vi "Save As DataTable.vi"(6 "overwrite file if exist (true)?":bool=TRUE, 8 "error in (no error)":errorcluster, 10 "filepath":path, 11 "JMP DataTable":refnum<k7>) -> (0 "error out":errorcluster, 3 "JMP data table out":refnum<k7>)   [LabVIEW 2019, in "JMP Automation.lvlib"]
doc: "save the data table at filepath. \n\nfilepath: path, including file name with the .jmp extention\noverwrite file if exist? if true, the the VI will overwrite an existing file"
uses:
  <instrlib>/LV_JMP_bridge/JMP Automation.lvlib
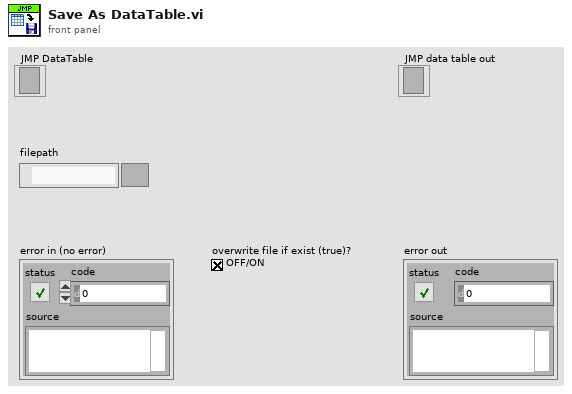
[diagram p1: front panel]
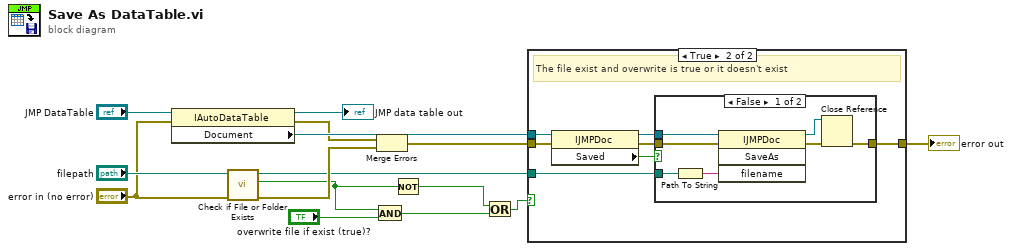
[diagram p0: block diagram]
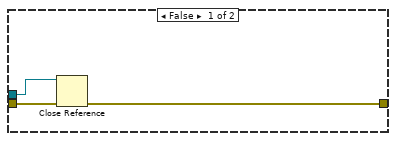
[diagram p2: hidden frame]
diagram:
  n1 = property class="IAutoDataTable"(reference="JMP DataTable", error in="error in (no error)") -> (reference out=→"JMP data table out":refnum<k7>, error out=w9:errorcluster, "Document"=w14:refnum<k7>)
  n2 = call <vilib>:"Check if File or Folder Exists.vi"("error in (no error)"="error in (no error)", "path"="filepath") -> ("error out"=w8:errorcluster, "file or folder exists?"=w2:bool, "dup path"=w7:path)  [unwired: 7 in]
  n3 = And(x=w2, y="overwrite file if exist (true)?") -> (x .and. y?=w3:bool)
  n4 = Merge Errors(w9, w8) -> (w6:errorcluster)
  n5 = Not(x=w2) -> (.not. x?=w4:bool)
  n6 = Or(x=w4, y=w3) -> (x .or. y?=w1:bool)
  n7 = case shown="True" w1 {
    tunnel: w14 -> [w18 w25]
    tunnel: [w17 w22] -> w12
    tunnel: w7 -> [_ w20]
    tunnel: w6 -> [w16 w19]
    frame False {
      n8 = Close Reference(reference=w18, error in (no error)=w16) -> (error out=w17:errorcluster)
    }
    frame True {
      # "The file exist and overwrite is true or it doesn't exist"
      n9 = property class="IJMPDoc"(reference=w25, error in=w19) -> (reference out=w23:refnum<k7>, error out=w21:errorcluster, "Saved"=w24:bool)
      n10 = case shown="False" w24 {
        tunnel: w23 -> [w32 _]
        tunnel: [w28 w33] -> w22
        tunnel: w21 -> [w27 w33]
        tunnel: w20 -> [w26 _]
        frame False {
          n11 = Path To String(path=w26) -> (string=w31:string)
          n12 = invoke class="IJMPDoc" method="SaveAs"(reference=w32, error in=w27, "filename"=w31) -> (reference out=w29:refnum<k7>, error out=w30:errorcluster)  [unwired: 1 in, 2 out]
          n13 = Close Reference(reference=w29, error in (no error)=w30) -> (error out=w28:errorcluster)
        }
        frame True {
        }
      }
    }
  }
  "error out" <- w12
